vi "Read module boolean values.vi"(9 "Label.Text":string="Phase Shift, deg", 11 "module ref":refnum<vi>) -> (2 "data":bool)   [LabVIEW 2017]
panel:
  out "Boolean Ref":refnum<vi>
  out "error out":errorcluster
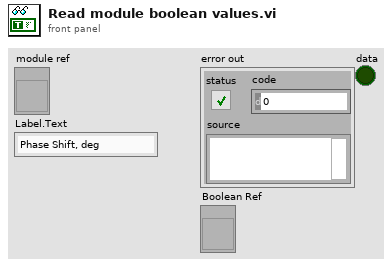
[diagram p1: front panel]
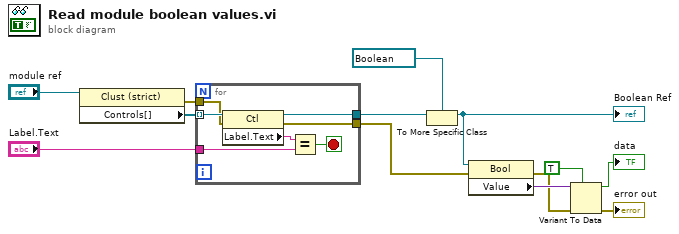
[diagram p0: block diagram]
diagram:
  n1 = property class="Clust (strict)"(reference="module ref") -> (error out=w3:errorcluster, "Controls[]"=w13:refnum<vi>[])  [unwired: 1 in, 1 out]
  n2 = for {
    tunnel: w13 -> [w20] mode=indexing
    tunnel: "Label.Text" -> [w19]
    tunnel: [w16] -> w11
    tunnel: w3 -> [w15]
    tunnel: [w14] -> w2
    stop <- w17 stop-if-true
    n3 = property class="Ctl"(reference=w20, error in=w15) -> (reference out=w16:refnum<vi>, error out=w14:errorcluster, "Label.Text"=w18:string)
    n4 = Equal?(x=w18, y=w19) -> (x = y?=w17:bool)
  }
  n5 = To More Specific Class(target class=refnum<vi> refnum ("Phase Shift, deg"), reference=w11) -> (specific class reference=w9:refnum<vi>)  [unwired: 1 in, 1 out]
  "Boolean Ref" <- w9
  n6 = property class="Bool"(reference=w9, error in=w2) -> (error out=w1:errorcluster, "Value"=w7:variant)  [unwired: 1 out]
  n7 = Variant To Data(error in=w1, type=TRUE, Variant=w7) -> (data=→"data":bool, error out=→"error out":errorcluster)
